vi "Right Shift.vi"(8 "Error In":errorcluster, 10 "x":i16, 11 "n":i16) -> (0 "Error Out":errorcluster, 3 "Value":i16)   [LabVIEW 2020, in "LiFingerprint.lvclass"]
uses:
  LiFingerprint.lvclass
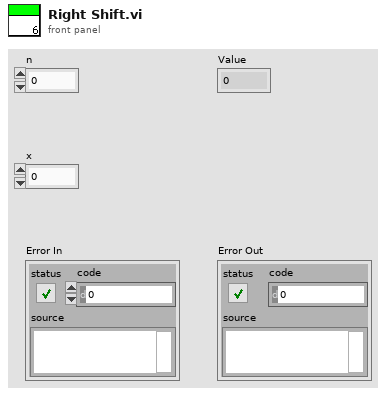
[diagram p1: front panel]
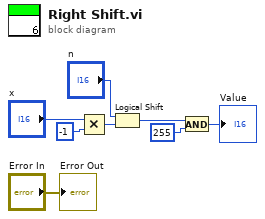
[diagram p0: block diagram]
diagram:
  n1 = Multiply(x="x", y=-1) -> (x*y=w4:i32)
  n2 = Logical Shift(y="n", x=w4) -> (x << y=w3:i32)
  n3 = And(x=w3, y=255) -> (x .and. y?=→"Value":i32)
  "Error Out" <- "Error In"
